vi "readFromXML.vi"(8 "error in (no error)":errorcluster, 10 "XML in":string, 11 "GuideTargetOffset in":refnum<class "GuideTargetOffset.lvclass">) -> (0 "error out":errorcluster, 3 "GuideTargetOffset out":refnum<class "GuideTargetOffset.lvclass">)   [LabVIEW 2022 SP3, in "TCSDataDefinitions.lvlib" / "TCSCommand.lvlib" / "OffsetCommands.lvlib" / "GuideTargetOffset.lvclass"]
uses:
  GuideTargetOffset.lvclass
  Offset/Offset.lvclass
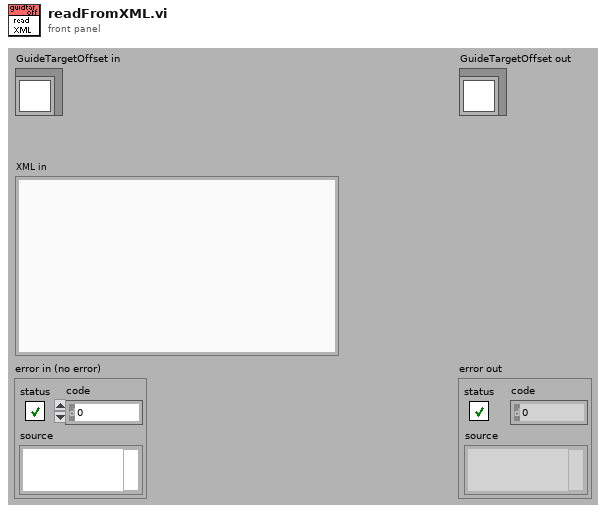
[diagram p1: front panel]
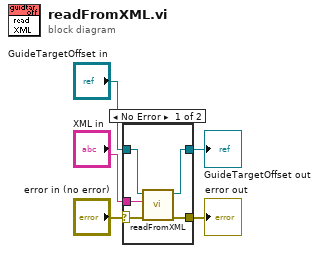
[diagram p0: block diagram]
diagram:
  n1 = case shown="No Error" "error in (no error)" {
    selector: "error in (no error)" -> [w8 w12]
    tunnel: [w7 w12] -> w4
    tunnel: [w9 w11] -> w2
    tunnel: "GuideTargetOffset in" -> [w10 w11]
    tunnel: "XML in" -> [w6 _]
    frame No Error {
      n2 = call-parent "readFromXML.vi"("error in (no error)"=w8, "XML in"=w6, "Offset in"=w10) -> ("error out"=w7:errorcluster, "Offset out"=w9:refnum<class "GuideTargetOffset.lvclass">)  [unwired: 7 out]
    }
    frame Error {
    }
  }
  "error out" <- w4
  "GuideTargetOffset out" <- w2
